vi "Manual Control - Connected Device Setup.vi"(8 "error in":errorcluster, 10 "DER_Info":T1, 11 "Master Controller in":refnum<class "EMS User Interface.lvclass">) -> (0 "error out":errorcluster, 3 "Master Controller out":refnum<class "EMS User Interface.lvclass">)   [LabVIEW 2018, in "EMS User Interface Actor.lvlib" / "EMS User Interface.lvclass"]
uses:
  EMS User Interface.lvclass
  <vilib>/ORNL/CSEISMIC DDS/CSEISMIC DDS Base/Data Types/DER_Info.ctl
  <vilib>/ORNL/CSEISMIC DDS/CSEISMIC DDS Base/Data Types/Controls/DeviceID.ctl
  EMS User Interface.lvclass/EMS User Interface.ctl
  <vilib>/ORNL/CSEISMIC DDS/CSEISMIC DDS Base/CSEISMIC DDS.lvclass
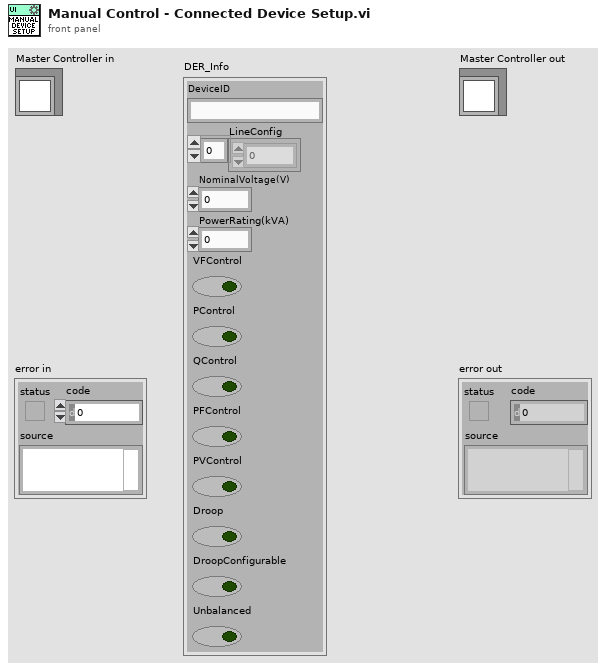
[diagram p1: front panel]
types:
  T1 = typedef "CSEISMIC DDS.lvlib/CSEISMIC DDS.lvclass/DER_Info.ctl" = cluster{"DeviceID":T2, "LineConfig":u8[], "NominalVoltage(V)":dbl, "PowerRating(kVA)":dbl, "VFControl":bool, "PControl":bool, "QControl":bool, "PFControl":bool, "PVControl":bool, "Droop":bool, "DroopConfigurable":bool, "Unbalanced":bool}
  T2 = typedef "CSEISMIC DDS.lvlib/CSEISMIC DDS.lvclass/DeviceID.ctl" = string
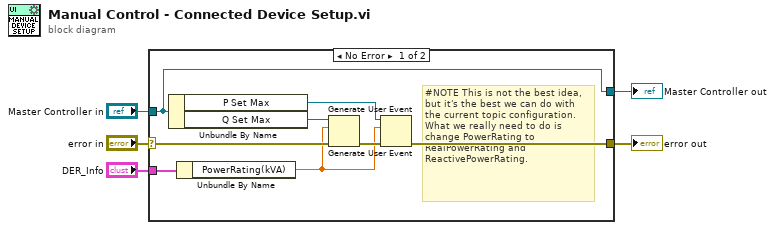
[diagram p0: block diagram]
diagram:
  n1 = case shown="No Error" "error in" {
    selector: "error in" -> [w12 w15]
    tunnel: [w10 w15] -> w4
    tunnel: [w13 w14] -> w2
    tunnel: "Master Controller in" -> [w13 w14]
    tunnel: "DER_Info" -> [w7 _]
    frame No Error {
      # "#NOTE This is not the best idea, but it's the best we can do with the current topic configuration. What we really need to do is change PowerRating to RealPowerRating and ReactivePowerRating."
      n2 = Unbundle By Name(w13) -> ("P Set Max"=w8:refnum<user-event>, "Q Set Max"=w9:refnum<user-event>)
      n3 = Unbundle By Name(w7) -> ("PowerRating(kVA)"=w6:dbl)
      n4 = Generate User Event(user event=w9, event data cluster=w6, error in=w12) -> (error out=w11:errorcluster)  [unwired: 1 in, 1 out]
      n5 = Generate User Event(user event=w8, event data cluster=w6, error in=w11) -> (error out=w10:errorcluster)  [unwired: 1 in, 1 out]
    }
    frame Error {
    }
  }
  "error out" <- w4
  "Master Controller out" <- w2
